vi "Lower Back Arms.vi"(8 "Abort":bool, 9 "Heightened Position":dbl=5.0, 10 "Lowered Position":dbl, 11 "Button":bool) -> (3 "Lower  Back Arms":bool)   [LabVIEW 2014]
uses:
  Lower Arm States.ctl
  Robot Global Data.vi
  Desired Arm Position.vi
panel:
  out "Start":bool
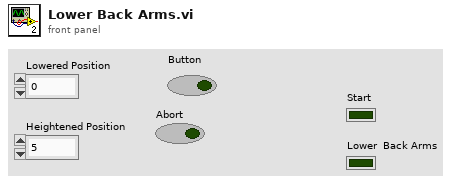
[diagram p1: front panel]
types:
  T1 = typedef "Lower Arm States.ctl" = enum16{"Start", "Lower + Open Back Arms", "Wait", "Close Arms + Lift"}
  T2 = typedef "WPI_DigitalInputDevRef.ctl" = cluster{"DevStatus":errorcluster, "DIO Channel":T3, "Controller":T4}
  T3 = typedef "FPGA_DIOChannel.ctl" = enum8{"DIO 0", "DIO 1", "DIO 2", "DIO 3", "DIO 4", "DIO 5", "DIO 6", "DIO 7", "DIO 8", "DIO 9", "DIO MXP 0", "DIO MXP 1", "DIO MXP 2", "DIO MXP 3", "DIO MXP 4", "DIO MXP 5", "DIO MXP 6", "DIO MXP 7", "DIO MXP 8", "DIO MXP 9", "DIO MXP 10", "DIO MXP 11", "DIO MXP 12", "DIO MXP 13", "DIO MXP 14", "DIO MXP 15", "Invalid"}
  T4 = typedef "FPGA_TypedefDigitalModule.ctl" = enum16{"Controller 1"}
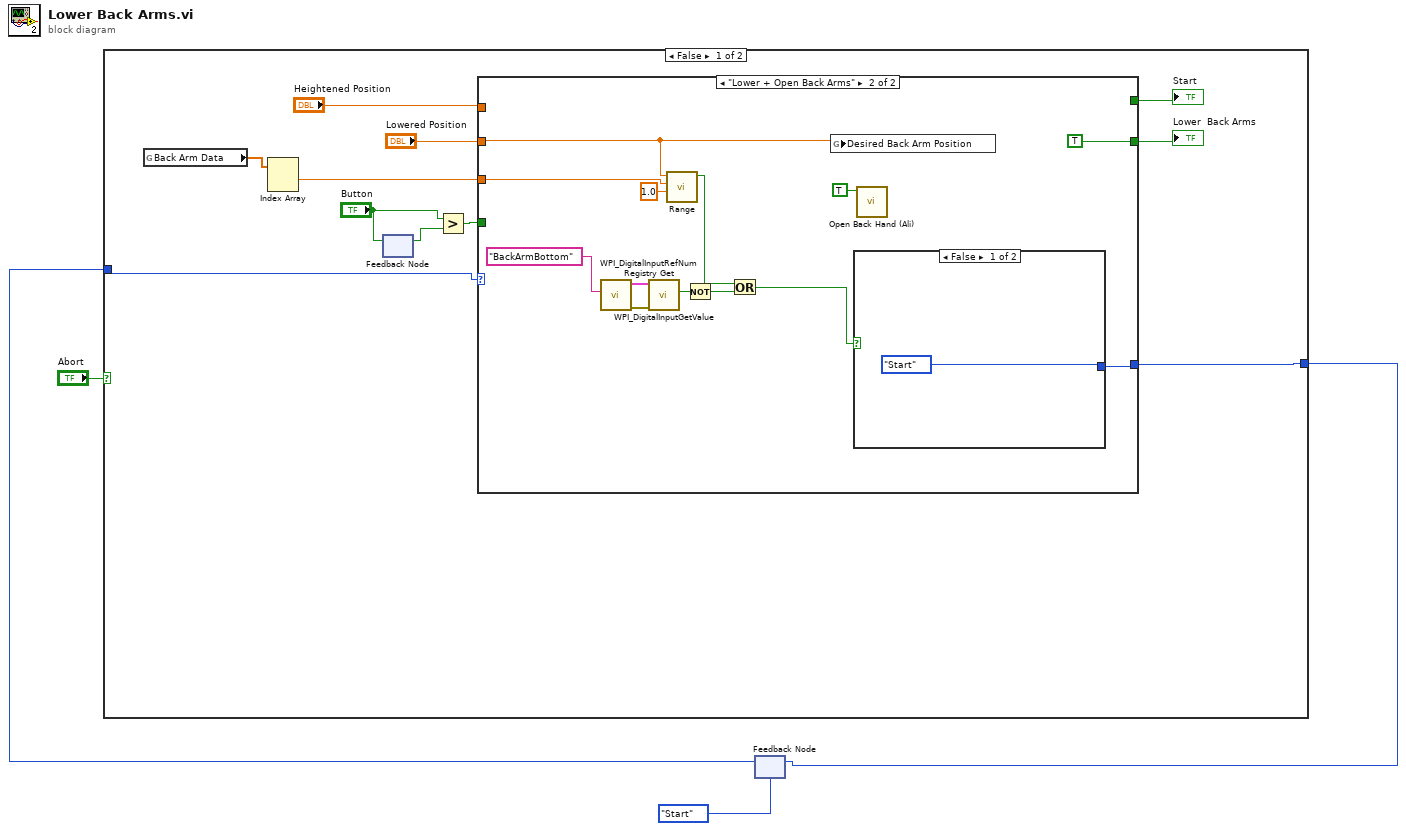
[diagram p0: block diagram]
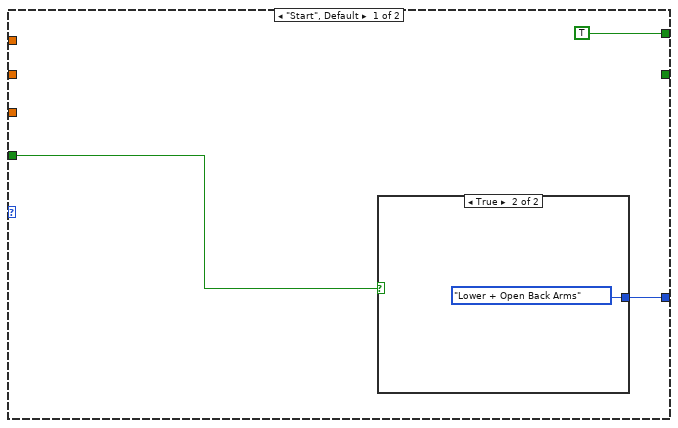
[diagram p2: hidden frame]
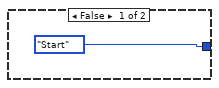
[diagram p3: hidden frame]
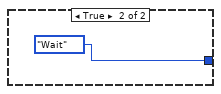
[diagram p4: hidden frame]
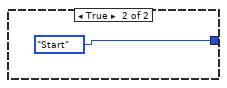
[diagram p5: hidden frame]
diagram:
  n1 = feedback #1(Lower_Arm_States."Start") -> (w1:T1)
  n2 = case shown="False" "Abort" {
    tunnel: [w8 Lower_Arm_States."Start"] -> w2
    tunnel: w1 -> [w7 _]
    frame False {
      n3 = global read "Robot Global Data.vi" "Back Arm Data"() -> (w11:dbl[])
      n4 = Index Array(array=w11) -> (element #1=w10:dbl)  [unwired: 2 in, 1 out]
      n5 = feedback #2() -> (w14:bool)  [unwired: 1 in]
      n6 = feedback-in #2("Button") -> ()
      n7 = Greater?(x="Button", y=w14) -> (0:w12:bool)
      n8 = case shown="\"Lower + Open Back Arms\"" w7 {
        tunnel: "Lowered Position" -> [_ w31]
        tunnel: w12 -> [w17 _]
        tunnel: [w18 w33] -> w8
        tunnel: w10 -> [_ w32]
        tunnel: "Heightened Position" -> [_ _]
        tunnel: [TRUE _] -> w6
        tunnel: [_ TRUE] -> w5
        frame "Start", Default {
          n9 = case shown="True" w17 {
            tunnel: [Lower_Arm_States."Start" Lower_Arm_States."Lower + Open Back Arms"] -> w18
            frame False {
            }
            frame True {
            }
          }
        }
        frame "Lower + Open Back Arms" {
          n10 = call <vilib>:"WPI_DigitalInputRefNum Registry Get.vi"("refnum name"="BackArmBottom") -> ("error out"=w29:errorcluster, "DigitalInputDevRef"=w28:T2)  [unwired: 9 in]
          n11 = call <vilib>:"WPI_DigitalInputGetValue.vi"("error in (no error)"=w29, "DigitalInputDevRef"=w28) -> ("Value"=w26:bool)  [unwired: 7 in, 2 out]
          n12 = call "Range.vi"("Range"=1.0, "Input"=w32, "In Range of"=w31) -> ("In Range?"=w27:bool)  [unwired: 8 in]
          n13 = Not(x=w26) -> (.not. x?=w22:bool)
          n14 = Or(x=w27, y=w22) -> (x .or. y?=w24:bool)
          n15 = global write "Desired Arm Position.vi" "Desired Back Arm Position"(w31) -> ()
          n16 = case shown="False" w24 {
            tunnel: [Lower_Arm_States."Start" Lower_Arm_States."Wait"] -> w33
            frame False {
            }
            frame True {
            }
          }
          n17 = call "Open Back Hand (Ali).vi"("Open?"=TRUE) -> ()  [unwired: 11 in]
        }
      }
      "Start" <- w6
      "Lower  Back Arms" <- w5
    }
    frame True {
    }
  }
  n18 = feedback-in #1(w2) -> ()
